vi "Get IC Array Size.vi"(8 "error in (no error)":errorcluster, 11 "PDE in":refnum<class "NI_PDE.lvclass">) -> (0 "error out":errorcluster, 2 "# of IC":i32, 3 "PDE out":refnum<class "NI_PDE.lvclass">)   [LabVIEW 2020, in "NI_PDE.lvlib" / "NI_PDE.lvclass"]
uses:
  <vilib>/gmath/pde.llb/PDEClass/NI_PDE.lvclass
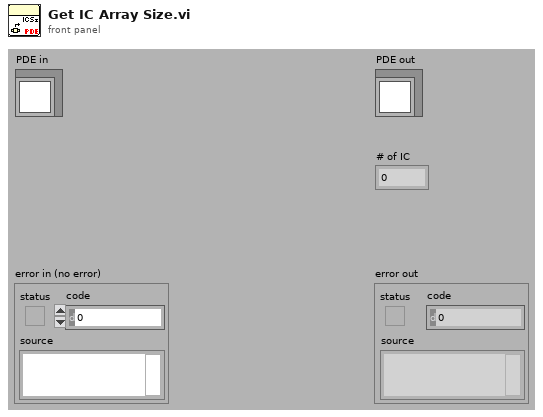
[diagram p1: front panel]
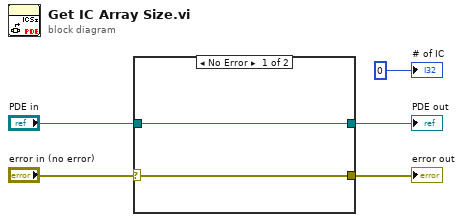
[diagram p0: block diagram]
diagram:
  n1 = case shown="No Error" "error in (no error)" {
    selector: "error in (no error)" -> [w6 w9]
    tunnel: "PDE in" -> [w7 w8]
    tunnel: [w7 w8] -> w4
    tunnel: [w6 w9] -> w3
    frame No Error {
    }
    frame Error {
    }
  }
  "PDE out" <- w4
  "error out" <- w3
  "# of IC" <- 0 ("# of IC")
